vi "SendMessageToMailbox.vi"(8 "error in (no error)":errorcluster, 10 "MailBoxMessage":refnum<class "MailBoxMessage.lvclass">, 11 "MailboxManager in":refnum<class "MailboxManager.lvclass">) -> (0 "error out":errorcluster, 3 "MailboxManager out":refnum<class "MailboxManager.lvclass">)   [LabVIEW 2020, in "MailboxManager.lvlib" / "MailboxManager.lvclass"]
uses:
  MailboxManager.lvclass
  MailBoxMessage/MailBoxMessage.lvclass
  C:/Program Files (x86)/National Instruments/LabVIEW 2020/vi.lib/ActorFramework/Message/Message.lvclass
  MailboxManager.lvclass/MailboxManager.ctl
  <vilib>/ActorFramework/Message Enqueuer/Message Enqueuer.lvclass/Message Enqueuer.ctl
  7106d21d-7aa8-4aaa-aea2-3e783fe011e8.vi
  <vilib>/ActorFramework/Message Priority Queue/Priority Enqueue.vi
  <vilib>/ActorFramework/Message Enqueuer/Message Enqueuer.lvclass
  C:/Users/taylo/Projects/LabVIEW/ActorMailbox/MailboxManager/MailBoxMessage/MailBoxMessage.lvclass
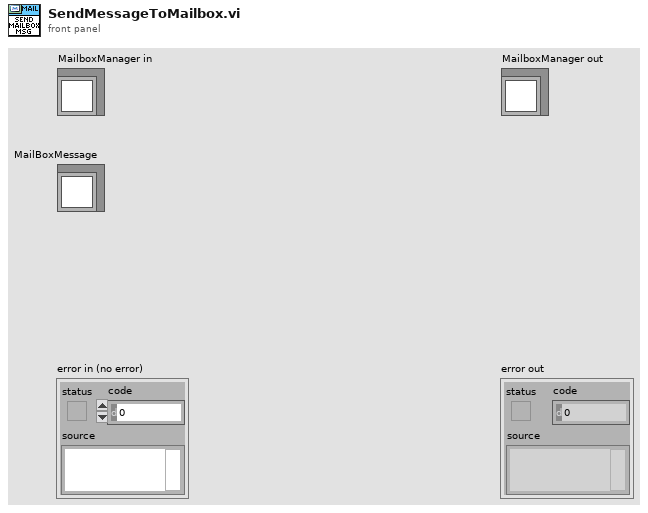
[diagram p1: front panel]
types:
  T1 = map{refnum<class "MailBoxMessage.lvclass">, refnum<class "Message Enqueuer.lvclass">[]}
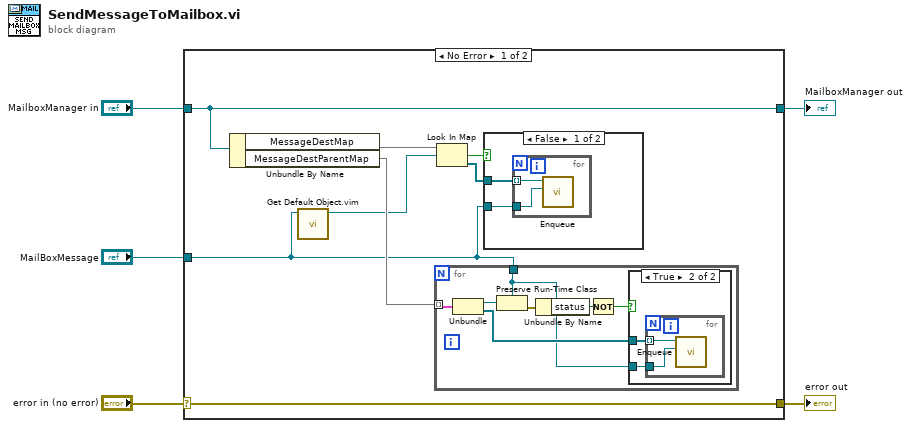
[diagram p0: block diagram]
diagram:
  n1 = case shown="No Error" "error in (no error)" {
    selector: "error in (no error)" -> [w13 w30]
    tunnel: [w13 w30] -> w4
    tunnel: [w12 w29] -> w2
    tunnel: "MailboxManager in" -> [w12 w29]
    tunnel: "MailBoxMessage" -> [w6 _]
    frame No Error {
      n2 = Unbundle By Name(w12) -> ("MessageDestMap"=w11:T1, "MessageDestParentMap"=w8:T1)
      n3 = call "Get Default Object.vim"("MailBoxMessage in"=w6) -> ("MailBoxMessage out"=w7:refnum<class "MailBoxMessage.lvclass">)  [unwired: 10 in]
      n4 = for {
        tunnel: w8 -> [w20] mode=indexing
        tunnel: w6 -> [w14]
        n5 = Unbundle(w20) -> ("MailBoxMessage"=w17:refnum<class "MailBoxMessage.lvclass">, "Message Enqueuers"=w15:refnum<class "Message Enqueuer.lvclass">[])
        n6 = Preserve Run-Time Class(object in=w17, 2:w14) -> (error out=w18:errorcluster)  [unwired: 1 in, 1 out]
        n7 = Unbundle By Name(w18) -> ("status"=w19:bool)
        n8 = Not(x=w19) -> (.not. x?=w16:bool)
        n9 = case shown="True" w16 {
          tunnel: w15 -> [_ w22]
          tunnel: w14 -> [_ w21]
          frame False {
          }
          frame True {
            n10 = for {
              tunnel: w22 -> [w24] mode=indexing
              tunnel: w21 -> [w23]
              n11 = call <vilib>:"Enqueue.vi"("Message"=w23, "Message Enqueuer in"=w24) -> ()  [unwired: 8 in, 2 out]
            }
          }
        }
      }
      n12 = Look In Map(map=w11, key=w7) -> (key not found?=w10:bool, value=w9:refnum<class "Message Enqueuer.lvclass">[])  [unwired: 1 in]
      n13 = case shown="False" w10 {
        tunnel: w9 -> [w26 _]
        tunnel: w6 -> [w25 _]
        frame False {
          n14 = for {
            tunnel: w26 -> [w28] mode=indexing
            tunnel: w25 -> [w27]
            n15 = call <vilib>:"Enqueue.vi"("Message"=w27, "Message Enqueuer in"=w28) -> ()  [unwired: 8 in, 2 out]
          }
        }
        frame True {
        }
      }
    }
    frame Error {
    }
  }
  "error out" <- w4
  "MailboxManager out" <- w2
